vi "Custom Error Handler.vi"(8 "error in (no error)":errorcluster={"status"=TRUE, "code"=122, "source"="yo yo!"}) -> (0 "error out":errorcluster)   [LabVIEW 2014, in "AvaSpec.lvlib"]
uses:
  AvaSpec.lvlib
  <vilib>/Utility/file.llb/Read From Spreadsheet File (string).vi
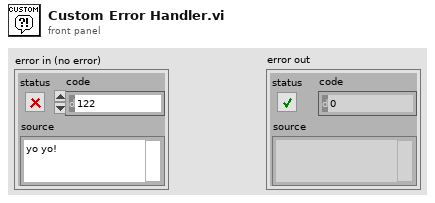
[diagram p1: front panel]
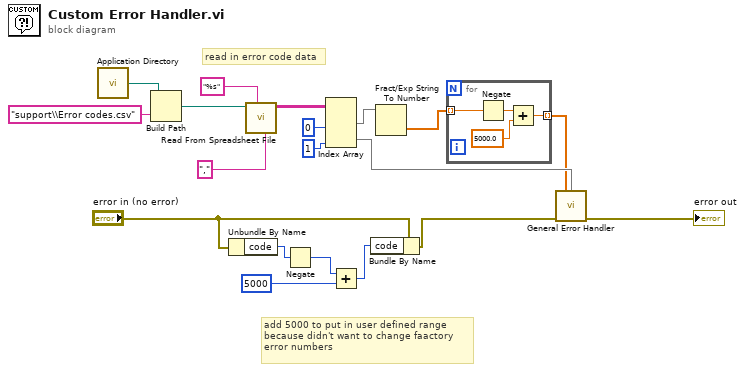
[diagram p0: block diagram]
diagram:
  # "read in error code data"
  # "add 5000 to put in user defined range\nbecause didn't want to change faactory\nerror numbers"
  n1 = call <vilib>:"Application Directory.vi"() -> ("Application Directory"=w3:path)
  n2 = Build Path(base path=w3, name or relative path="support\\Error codes.csv") -> (appended path=w1:path)
  n3 = Unbundle By Name("error in (no error)") -> ("code"=w5:i32)
  n4 = call-poly <vilib>:"Read From Spreadsheet File.vi"("delimiter (\\t)"="," ("delimiter (\\t)"), "format (%s)"="%s" ("format (%.3f)"), "file path (dialog if empty)"=w1) -> ("all rows"=w16:string[][])  [unwired: 4 in, 4 out]
  n5 = Negate(x=w5) -> (-x=w4:i32)
  n6 = Index Array(array=w16, index (col) #1=0 ("disabled index (col)"), index (col) #2=1 ("index (col)")) -> (element #1=w13:string[], element #2=w12:string[])  [unwired: 2 in]
  n7 = Add(x=w4, y=5000) -> (x+y=w9:i32)
  n8 = Bundle By Name(cluster="error in (no error)", "code"=w9) -> (w10:errorcluster)
  n9 = Fract/Exp String To Number(string=w13) -> (number=w8:dbl[])  [unwired: 3 in, 1 out]
  n10 = for {
    tunnel: w8 -> [w20] mode=indexing
    tunnel: [w22] -> w7 mode=indexing
    n11 = Negate(x=w20) -> (-x=w21:dbl)
    n12 = Add(x=w21, y=5000.0) -> (x+y=w22:dbl)
  }
  n13 = call <vilib>:"General Error Handler.vi"("[user-defined codes]"=w7, "[user-defined descriptions]"=w12, "error in (no error)"=w10) -> ("error out"=→"error out":errorcluster)  [unwired: 8 in, 4 out]
